vi "DB - [Config].[SoftwareSolution].vi"(4 "[LanguageId]":string="en", 5 "Application":string, 6 "[PlantId]":string="4070", 7 "DB Connection":T2={"Open"=TRUE, "Close"=TRUE}, 8 "error in (no error)":errorcluster, 11 "connection reference":T1) -> (0 "SUMMARY":errorcluster, 1 "1D data":string[](array[string]), 3 "connection reference":T1)   [LabVIEW 2013]
doc: "USE [<DB>]\nSELECT \n a.[LogoFile]\n ,a.[TimeZone]\n ,CAST(c.[SolutionName] AS varbinary(max)) AS [Title Of Application]\n ,b.[FileServerPath] \n ,b.[ClientFilePath]\n ,b.[CmsServerTz] AS [CSM Server TimeZone]\n ,a.[SoftwareSolutionId]\nFROM [Config].[Plant] AS a\nJOIN [Config].[SoftwareSolution] AS b\nON \n a.[PlantId] = b.[PlantId] AND\n a.[SoftwareSolutionId] = b.[SoftwareSolutionId] \nJOIN [Config].[Solution] as c\nON b.[SolutionId] = c.[SolutionId]\n\nWHERE a.[PlantId] = '4070' AND a.[Inactive] = '0' AND b.[Inactive] = '0' AND c.[LanguageId] = 'en' AND c.[Inactive] = '0'"
uses:
  <vilib>/addons/database/Connection.llb/Conn ObjectReference.ctl
  Controls/DB - OpenClose.ctl
  Controls/Global SRTRS.vi
  Controls/Global CMS.vi
  Controls/Global AMS.vi
  <vilib>/addons/database/Connection.llb/Conn Execute.vi
  <vilib>/addons/database/Recordset.llb/Rec Fetch Recordset Data (R).vi
  <vilib>/addons/database/Recordset.llb/Rec Destroy - Connection.vi
  <vilib>/addons/database/Connection.llb/DB Tools Open Connec (String).vi
  <vilib>/addons/database/_DB Variant To Data/Database Variant To Data.xnode
  <vilib>/addons/database/NI_Database_API.lvlib
panel:
  out "DB.Config.Solution":string="SRTRS.Config.SoftwareSolution"
  out "Close":errorcluster
  out "SQL Statement":string
  out "2D data (NA)":string[][](array[string])
  out "DB.Config.SoftwareSolution":string="SRTRS.Config.SoftwareSolution"
  out "DB.Config.Plant":string="SRTRS.Config.Plant"
  out "Connection Information":T3={"Connection "="SQL Server 32bit HPEnvy", "Username"="admin", "Password"="admin123"}
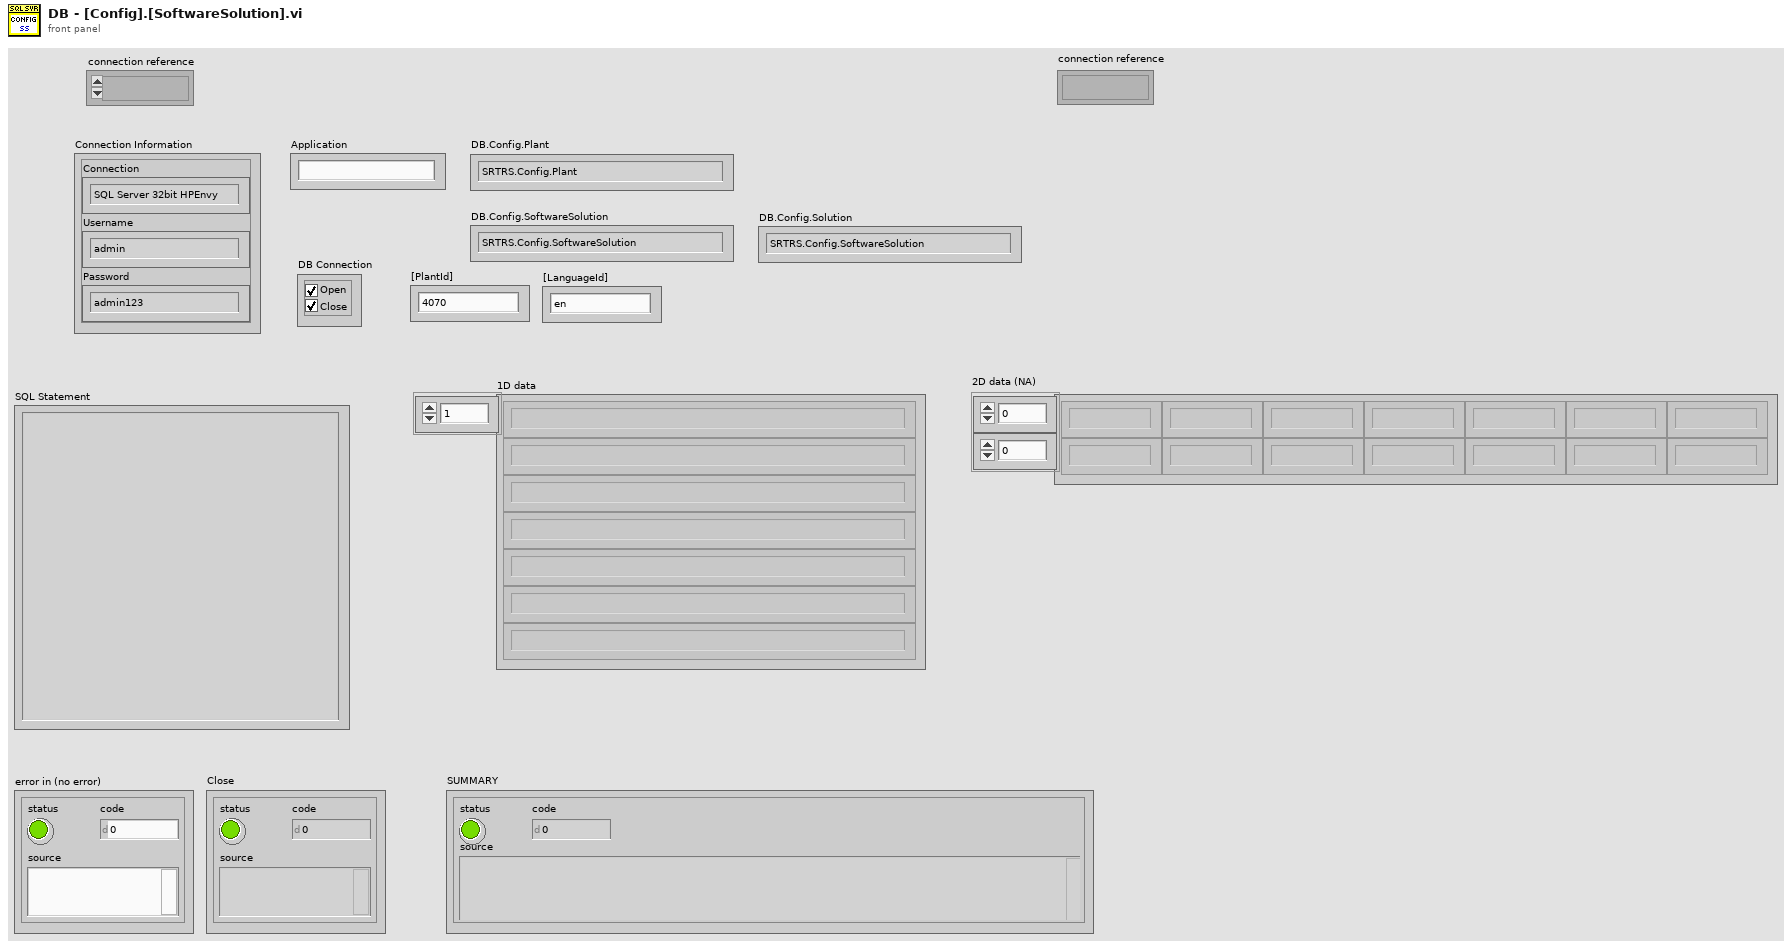
[diagram p1: front panel]
types:
  T1 = typedef "NI_Database_API.lvlib/Conn ObjectReference.ctl" = refnum<k1>
  T2 = typedef "DB - OpenClose.ctl" = cluster{"Open":bool, "Close":bool}
  T3 = cluster{"Connection ":string, "Username":string, "Password":string}
  T4 = typedef "Enum - InteractiveMode-SubVIMode.ctl" = enum16{"Interactive", "subVI Mode"}
  T5 = typedef "Connection Information Cluster.ctl" = cluster{"Connection ":string, "Username":string, "Password":string}
  T6 = typedef "DB - DB.Schema.Table.ctl" = cluster{"DB":string, "Schema":string, "Table":string}
  T7 = typedef "NI_Database_API.lvlib/Rec ObjectReference.ctl" = refnum<k1>
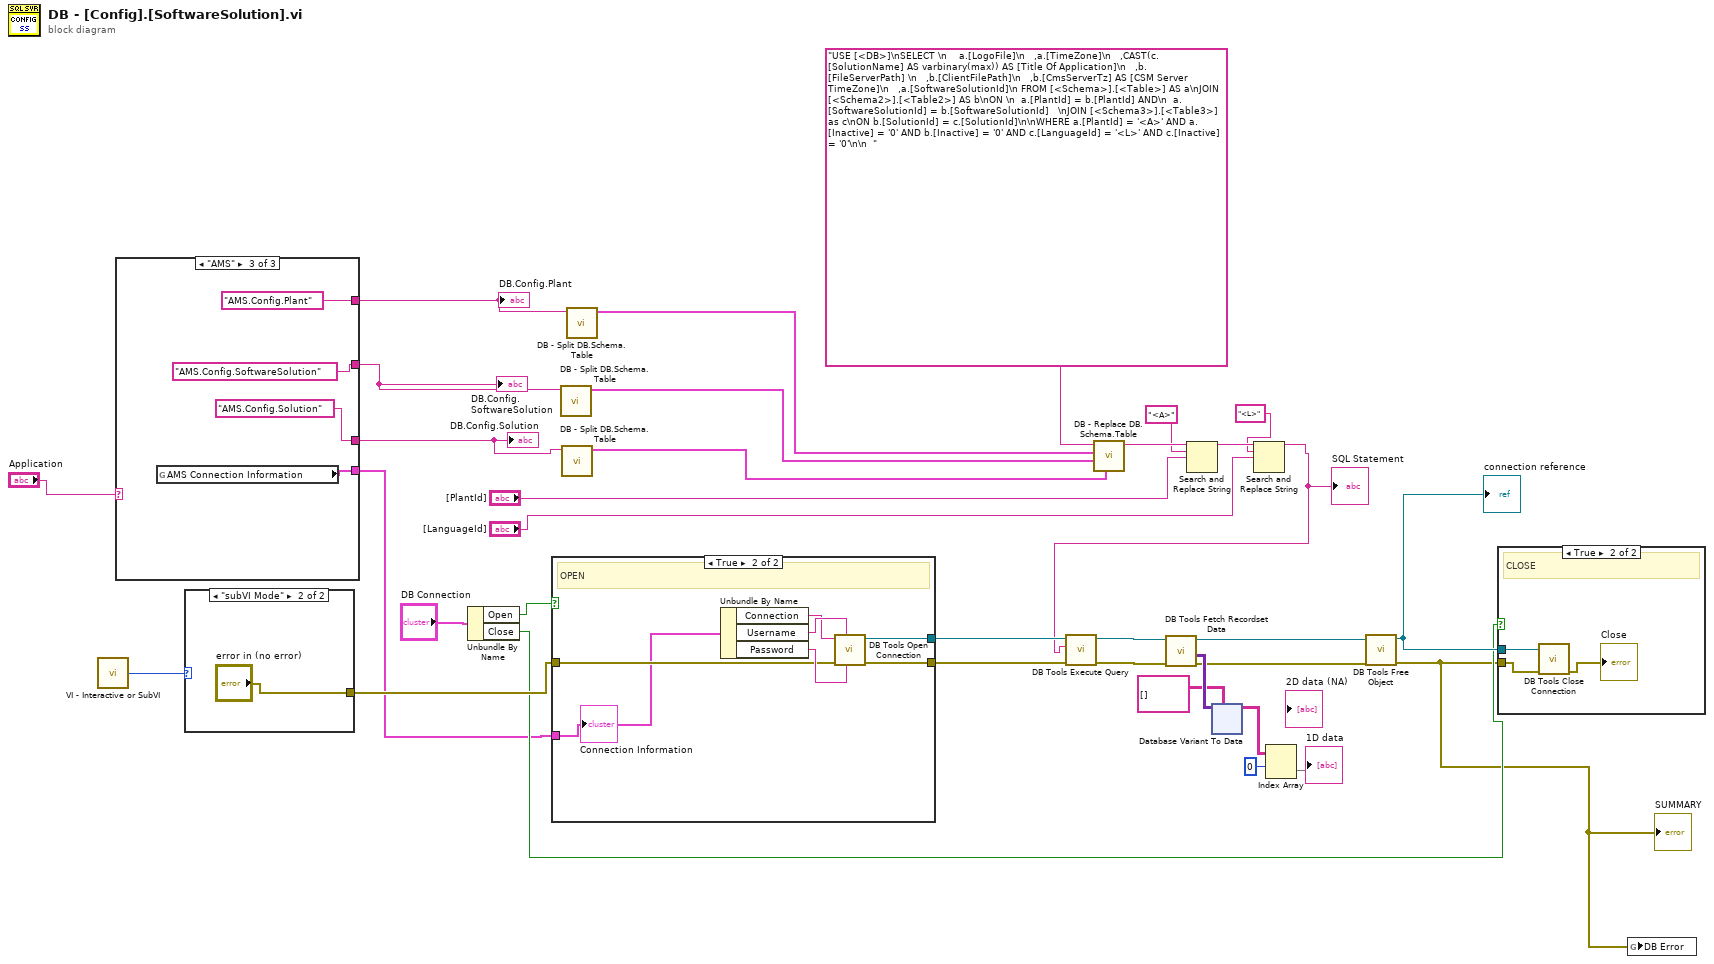
[diagram p0: block diagram]
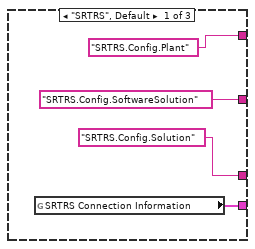
[diagram p2: hidden frame]
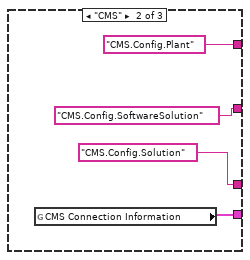
[diagram p3: hidden frame]
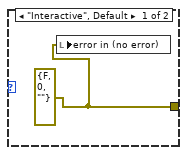
[diagram p5: hidden frame]
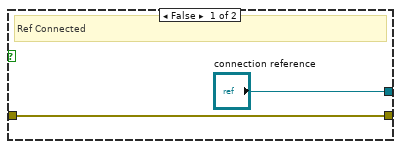
[diagram p6: hidden frame]
diagram:
  n1 = call "VI - Interactive or SubVI.vi"() -> ("Mode"=w32:T4)  [unwired: 5 in]
  n2 = case shown="\"AMS\"" "Application" {
    tunnel: [w38 w42 w43] -> w9
    tunnel: ["SRTRS.Config.Plant" ("DB.Schema.Table\nSRTRS.Config.Plant") "CMS.Config.Plant" ("DB.Schema.Table\nSRTRS.Config.Plant") "AMS.Config.Plant" ("DB.Schema.Table\nSRTRS.Config.Plant")] -> w8
    tunnel: ["SRTRS.Config.SoftwareSolution" ("DB.Schema.Table \nSRTRS.Config.SoftwareSolution") "CMS.Config.SoftwareSolution" ("DB.Schema.Table \nSRTRS.Config.SoftwareSolution") "AMS.Config.SoftwareSolution" ("DB.Schema.Table \nSRTRS.Config.SoftwareSolution")] -> w7
    tunnel: ["SRTRS.Config.Solution" ("DB.Schema.Table \nSRTRS.Config.SoftwareSolution") "CMS.Config.Solution" ("DB.Schema.Table \nSRTRS.Config.SoftwareSolution") "AMS.Config.Solution" ("DB.Schema.Table \nSRTRS.Config.SoftwareSolution")] -> w6
    frame "SRTRS", Default {
      n3 = global read "Global SRTRS.vi" "SRTRS Connection Information"() -> (w38:T5)
    }
    frame "CMS" {
      n4 = global read "Global CMS.vi" "CMS Connection Information"() -> (w42:T5)
    }
    frame "AMS" {
      n5 = global read "Global AMS.vi" "AMS Connection Information"() -> (w43:T5)
    }
  }
  "DB.Config.Plant" <- w8
  "DB.Config.SoftwareSolution" <- w7
  "DB.Config.Solution" <- w6
  n6 = case shown="\"subVI Mode\"" w32 {
    tunnel: [w47 "error in (no error)"] -> w31
    frame "Interactive", Default {
      w47 = errorcluster {"status"=FALSE, "code"=0, "source"=""} ("error in (no error)")
      n7 = local write "error in (no error)"(w47) -> ()
    }
    frame "subVI Mode" {
    }
  }
  n8 = Unbundle By Name("DB Connection") -> ("Open"=w33:bool, "Close"=w21:bool)
  n9 = case shown="True" w33 {
    tunnel: ["connection reference" w54] -> w24
    tunnel: w31 -> [w49 w53]
    tunnel: [w49 w52] -> w23
    tunnel: w9 -> [_ w51]
    frame False {
      # "Ref Connected"
    }
    frame True {
      # "OPEN"
      n10 = Unbundle By Name(w51) -> ("Connection"=w56:string, "Username"=w57:string, "Password"=w55:string)
      n11 = call-poly <vilib>:"DB Tools Open Connection.vi"("password"=w55, "userID"=w57, "error in (no error)"=w53, "connection information"=w56) -> ("error out"=w52:errorcluster, "connection reference"=w54:T1)  [unwired: 4 in]
      "Connection Information" <- w51
    }
  }
  n12 = call "DB - Split DB.Schema.Table.vi"("DB.Schema.Table"=w7) -> ("DB.Schema.Table"=w15:T6)  [unwired: 10 in]
  n13 = call "DB - Split DB.Schema.Table.vi"("DB.Schema.Table"=w6) -> ("DB.Schema.Table"=w5:T6)  [unwired: 10 in]
  n14 = call "DB - Split DB.Schema.Table.vi"("DB.Schema.Table"=w8) -> ("DB.Schema.Table"=w20:T6)  [unwired: 10 in]
  n15 = call "DB - Replace DB.Schema.Table.vi"("DB.Schema.Table 3"=w5, "DB.Schema.Table 2"=w15, "DB.Schema.Table"=w20, "string in"="USE [<DB>]\nSELECT \n    a.[LogoFile]\n   ,a.[TimeZone]\n   ,CAST(c.[SolutionName] AS varbinary(max)) AS [Title Of Application]\n   ,b.[FileServerPath] \n   ,b.[ClientFilePath]\n   ,b.[CmsServerTz] AS [CSM Server TimeZone]\n   ,a.[SoftwareSolutionId]\n FROM [<Schema>].[<Table>] AS a\nJOIN [<Schema2>].[<Table2>] AS b\nON \n  a.[PlantId] = b.[PlantId] AND\n  a.[SoftwareSolutionId] = b.[SoftwareSolutionId]   \nJOIN [<Schema3>].[<Table3>] as c\nON b.[SolutionId] = c.[SolutionId]\n\nWHERE a.[PlantId] = '<A>' AND a.[Inactive] = '0' AND b.[Inactive] = '0' AND c.[LanguageId] = '<L>' AND c.[Inactive] = '0'\n\n  ") -> ("string out"=w18:string)  [unwired: 6 in, 1 out]
  n16 = Search and Replace String(input string=w18, search string="<A>", replace string="[PlantId]") -> (result string=w3:string)  [unwired: 5 in, 3 out]
  n17 = Search and Replace String(input string=w3, search string="<L>", replace string="[LanguageId]") -> (result string=w4:string)  [unwired: 5 in, 3 out]
  "SQL Statement" <- w4
  n18 = call-poly <vilib>:"DB Tools Execute Query.vi"("error in (no error)"=w23, "SQL query"=w4, "connection reference"=w24) -> ("error out"=w30:errorcluster, "recordset reference"=w29:T7)  [unwired: 5 in]
  n19 = call-poly <vilib>:"DB Tools Fetch Recordset Data.vi"("error in (no error)"=w30, "recordset reference"=w29) -> ("error out"=w25:errorcluster, "recordset data"=w28:variant[][], "recordset reference out"=w26:T7)  [unwired: 3 in]
  n20 = xnode "Database Variant To Data"("database variant"=w28, "type"=string[][] []) -> ("data"=w14:string[][])  [unwired: 1 in, 1 out]
  n21 = Index Array(array=w14, index (row)=0) -> (element=→"1D data":string[])  [unwired: 1 in]
  n22 = call-poly <vilib>:"DB Tools Free Object.vi"("error in (no error)"=w25, "recordset reference"=w26) -> ("error out"=w11:errorcluster, "connection reference"=w22:T1)  [unwired: 8 in]
  "SUMMARY" <- w11
  "connection reference" <- w22
  n23 = case shown="True" w21 {
    tunnel: w22 -> [_ w60]
    tunnel: w11 -> [_ w59]
    frame False {
      # "Ref Connected"
    }
    frame True {
      # "CLOSE"
      n24 = call <vilib>:"DB Tools Close Connection.vi"("error in (no error)"=w59, "connection reference"=w60) -> ("error out"=→"Close":errorcluster)  [unwired: 5 in]
    }
  }
  n25 = global write "Global SRTRS.vi" "DB Error"(w11) -> ()
